vi "TCP HeartBeat Generator.vi"() -> ()   [LabVIEW 2019, in "Common System Tests.lvclass"]
uses:
  Common System Tests.lvclass
panel:
  in  "HeartBeat Period (s)":dbl=10.0 format="%#_13g"
  out "HeartBeat Array":string[](array[string])
  out "bytes written":i32
  in  "HeartBeat Content":string
  in  "error in (no error)":errorcluster
  out "error out":errorcluster
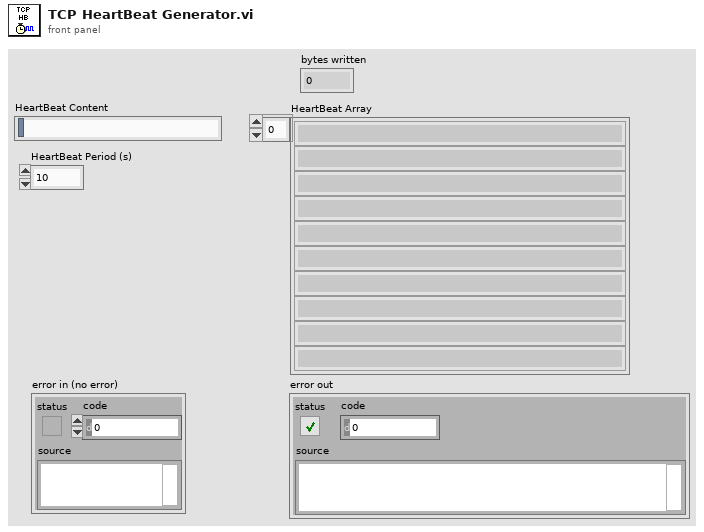
[diagram p1: front panel]
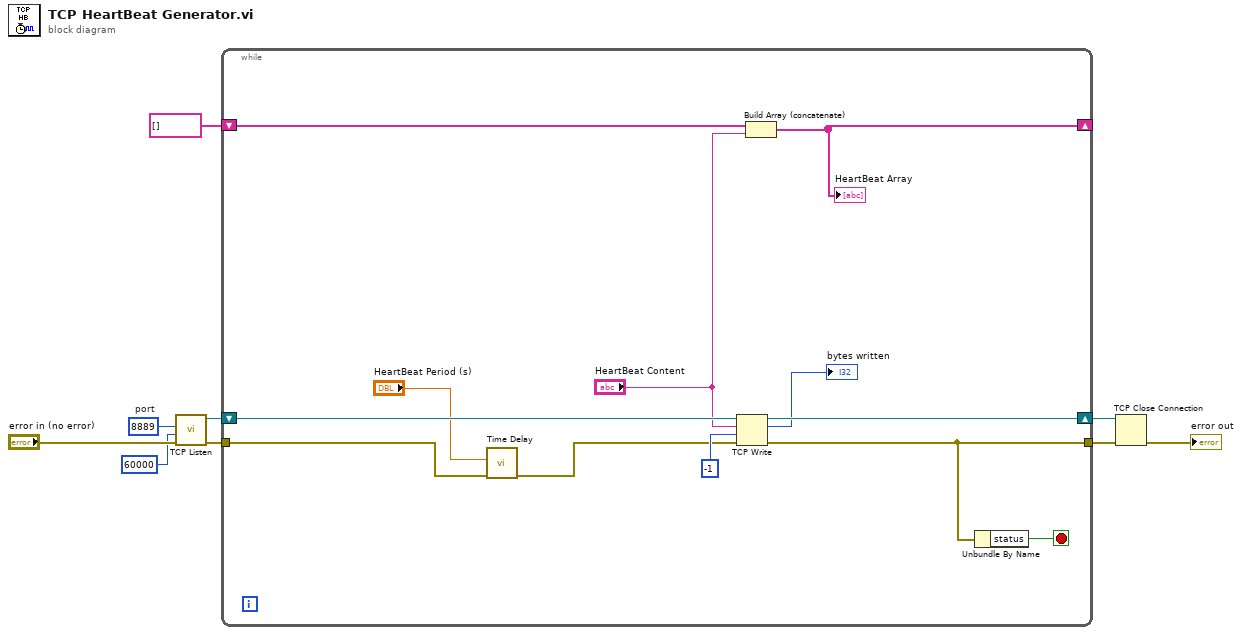
[diagram p0: block diagram]
diagram:
  w6 = u16 8889  # port
  n1 = call <vilib>:"TCP Listen.vi"("error in (no error)"="error in (no error)", "timeout ms (wait forever: -1)"=60000, "port"=w6) -> ("error out"=w4:errorcluster, "connection ID"=w5:refnum<k5>)  [unwired: 4 in, 3 out]
  n2 = while {
    shift-right: [w16] -> _
    shift-left: string[] [] -> [w20]
    shift-right: [w17] -> w9
    shift-left: w5 -> [w21]
    tunnel: w4 -> [w10]
    tunnel: [w18] -> w8
    stop <- w19 stop-if-true
    n3 = call "Time Delay"("error in (no error)"=w10, "Delay Time (s)"="HeartBeat Period (s)") -> ("error out"=w11:errorcluster)  [unwired: 9 in]
    n4 = TCP Write(connection ID=w21, data in="HeartBeat Content", error in (no error)=w11, 9:-1 ("timeout ms (25000)")) -> (connection ID out=w17:refnum<k5>, bytes written=→"bytes written":i32, error out=w18:errorcluster)
    n5 = Build Array (concatenate)(w20, "HeartBeat Content") -> (w16:string[])
    "HeartBeat Array" <- w16
    n6 = Unbundle By Name(w18) -> ("status"=w19:bool)
  }
  n7 = TCP Close Connection(connection ID=w9, error in (no error)=w8) -> (error out=→"error out":errorcluster)  [unwired: 1 in, 1 out]
